vi "RoboMovement_WithIR.vi"() -> ()   [LabVIEW 2020]
uses:
  <vilib>/Instr/_visa.llb/VISA Configure Serial Port (Instr).vi
panel:
  out "Indicator 3":bool
  out "Indicator 2":string
  in  "stop 2":bool
  out "read buffer":string
  in  "VISA resource name":refnum<visa-resource-name>="COM3"
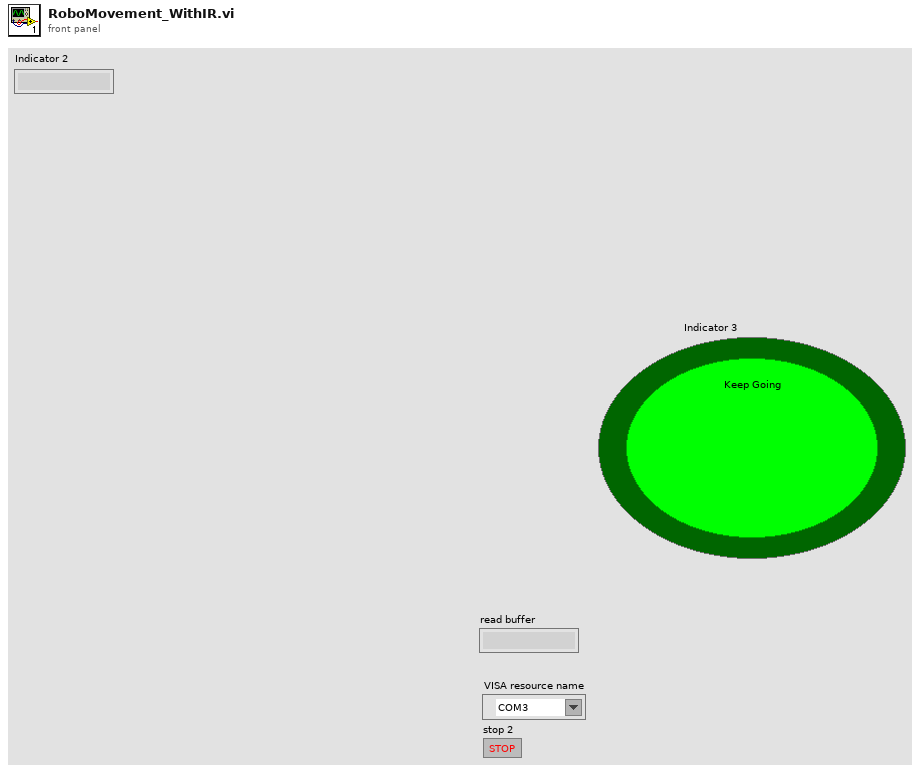
[diagram p1: front panel]
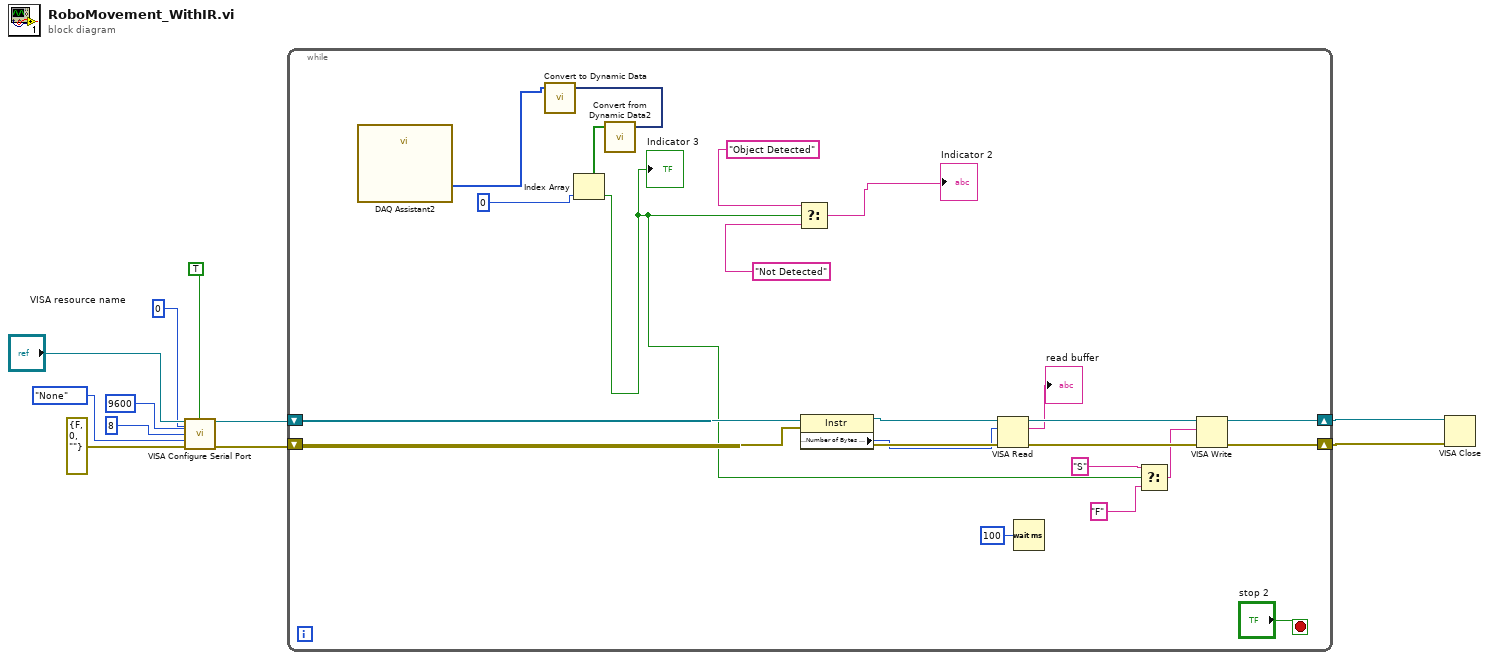
[diagram p0: block diagram]
diagram:
  n1 = call-poly "VISA Configure Serial Port"("VISA resource name"="VISA resource name", "termination char\n(0xA = '\\n' = LF)"=u8 0 ("termination char\n(0xA = '\\n' = LF)"), "Enable Termination\nChar (T)"=TRUE ("Enable Termination\nChar (T)"), "baud rate (9600)"=u32 9600, "data bits (8)"=u16 8, "parity (0:none)"=enum16{"None", "Odd", "Even", "Mark", "Space"}."None", "error in (no error)"=errorcluster {"status"=FALSE, "code"=0, "source"=""}) -> ("VISA resource name out"=w4:refnum<visa-resource-name>, "error out"=w2:errorcluster)  [unwired: 7 in]
  n2 = while {
    shift-right: [w31] -> w3
    shift-left: w4 -> [w34]
    shift-right: [w27] -> w1
    shift-left: w2 -> [w30]
    stop <- "stop 2" stop-if-true
    n3 = call "DAQ Assistant2"() -> ("data"=w13:u32[])  [unwired: 17 in, 2 out]
    n4 = call "Convert to Dynamic Data"("Array"=w13) -> ("Dynamic Data Type"=w15:dynamicdata)  [unwired: 3 in]
    n5 = call "Convert from Dynamic Data2"("Dynamic Data Type"=w15) -> ("Array"=w14:bool[])  [unwired: 3 in]
    n6 = Index Array(array=w14, index=0) -> (element=w12:bool)
    "Indicator 3" <- w12
    n7 = Select(t="Object Detected", s=w12, f="Not Detected") -> (s? t:f=→"Indicator 2":string)
    n8 = property class="Instr"(reference=w34, error in=w30) -> (reference out=w33:refnum<visa-resource-name>, error out=w29:errorcluster, "Serial Settings:Number of Bytes at Serial Port"=w24:u32)
    n9 = VISA Read(VISA resource name=w33, byte count=w24, error in (no error)=w29) -> (VISA resource name out=w32:refnum<visa-resource-name>, read buffer=→"read buffer":string, error out=w28:errorcluster)  [unwired: 1 out]
    n10 = Wait (ms)(milliseconds to wait=u32 100) -> ()  [unwired: 1 out]
    n11 = Select(t="S", s=w12, f="F") -> (s? t:f=w20:string)
    n12 = VISA Write(VISA resource name=w32, write buffer=w20, error in (no error)=w28) -> (VISA resource name out=w31:refnum<visa-resource-name>, error out=w27:errorcluster)  [unwired: 1 out]
  }
  n13 = VISA Close(VISA resource name=w3, error in (no error)=w1) -> ()  [unwired: 1 out]
